vi "字符串转unicode.vi"(0 "ASCII string":string caption="ASCII字符串") -> (1 "unicode string":string caption="unicode字符串", 2 "交换高低字节":string)   [LabVIEW 2013]
panel:
  # "ATK-SIM900A中英文短信发送测试"
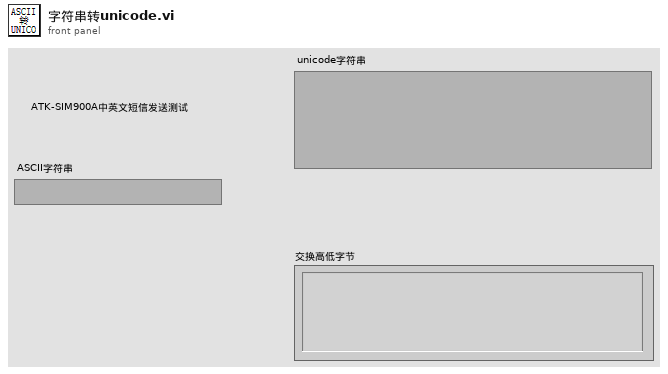
[diagram p1: front panel]
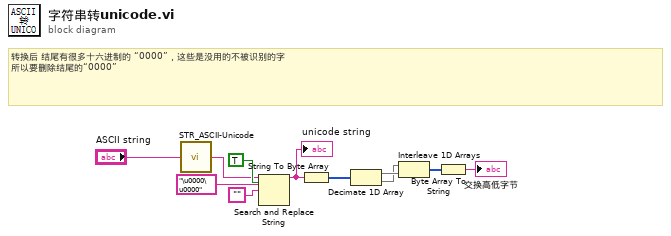
[diagram p0: block diagram]
diagram:
  # "转换后 结尾有很多十六进制的 “0000”，这些是没用的不被识别的字\n所以要删除结尾的“0000”"
  n1 = call <vilib>:"STR_ASCII-Unicode.vi"("ASCII string"="ASCII string") -> ("unicode string"=w3:string)
  n2 = Search and Replace String(replace all?=TRUE ("替换全部？(F)"), input string=w3, search string="\u0000\u0000" ("搜索字符串"), replace string="") -> (result string=w1:string)  [unwired: 4 in, 3 out]
  "unicode string" <- w1
  n3 = String To Byte Array(string=w1) -> (unsigned byte array=w7:u8[])
  n4 = Decimate 1D Array(w7) -> (w10:u8[], w9:u8[])
  n5 = Interleave 1D Arrays(w9, w10) -> (w8:u8[])
  n6 = Byte Array To String(unsigned byte array=w8) -> (string=→"交换高低字节":string)
